vi "Color Table Generator.vi"() -> (0 "Color Map":u32[](array[colorbox])=[0, 15606540, 15541260, 15410444, 15345165, 15279629, 15214349, 15083534, 15018254, 14952974, 14822158, 14756622, 14691343, 14560527, 14495247, 14429968, 14364688, 14233616, 14168336, 14103056, 13972241, 13906961, 13841681, 13776146, 13645330, 13580050, 13514770, 13383954, 13318675, 13253395, 13122323, 13057044, 12991764, 12926484, 12795668, 12730388, 12664853, 12534037, 12468757, 12403478, 12338198, 12207382, 12141846, 12076566, 11945751, 11880471, 11815191, 11749912, 11618840, 11553560, 11488280, 11357464, 11292185, 11226905, 11096089, 11030554, 10965274, 10899994, 10769178, 10703898, 10638619, 10507547, 10442267, 10376988, 10311708, 10180892, 10115612, 10050076, 9919261, 9853981, 9788701, 9657886, 9592606, 9527070, 9461790, 9330974, 9265695, 9200415, 9069599, 9004064, 8938784, 8873504, 8742688, 8677408, 8612129, 8481313, 8415777, 8350498, 8219682, 8154402, 8089122, 8023842, 7892771, 7827491, 7762211, 7631396, 7566116, 7500836, 7435300, 7304484, 7239205, 7173925, 7043109, 6977830, 6912294, 6847014, 6716198, 6650918, 6585639, 6454823, 6389543, 6324008, 6193192, 6127912, 6062632, 5997352, 5866537, 5801001, 5801257, 5735978, 5736234, 5670954, 5671210, 5605674, 5605931, 5540651, 5540907, 5475628, 5475884, 5410348, 5410605, 5345327, 5345584, 5279793, 5279539, 5213748, 5213493, 5147703, 5147704, 5081913, 5081659, 5015868, 5015613, 4949823, 4949568, 4949314, 4883523, 4883268, 4817734, 4817479, 4751688, 4751434, 4685643, 4685388, 4619598, 4619343, 4553552, 4553298, 4487763, 4487508, 4421718, 4421463, 4355672, 4355418, 4289627, 4289372, 4223582, 4223327, 4157792, 4157538, 4091747, 4091492, 4091238, 4025447, 4025192, 3959402, 3959147, 3893357, 3893358, 3827567, 3827313, 3761522, 3761267, 3695477, 3695222, 3629431, 3629177, 3563386, 3563387, 3497597, 3497342, 3431551, 3431297, 3365506, 3365251, 3299461, 3299206, 3233415, 3233161, 3167626, 3167371, 3167117, 3101326, 3101071, 3035281, 3035026, 2969235, 2968981, 2903190, 2903192, 2837401, 2837146, 2771356, 2771101, 2705310, 2705056, 2639265, 2639010, 2573220, 2573221, 2507430, 2507176, 2441385, 2441130, 2375340, 2375085, 2309294, 2309040, 2308785, 2243250, 2242996, 2177205, 2176950, 2111160, 2110905, 2045114, 2044860, 1979069, 1978814, 1913280, 1913025, 1847235, 1846980, 1781189, 1780935, 1715144, 1714889, 1649099, 1648844, 1583309, 1583055, 1517264, 1517009, 1451219, 1450964, 16711680])   [LabVIEW 2013]
doc: "Color Table Generator.vi is a subVI called by Color Table Example.vi\n\nThis VI generates a color table based on the beginning, middle, and end RGB color combinations the user specifies. Using an XY graph and cursors, the user mixes red, green, and blue components to create the start, middle, and end color combinations for the color table."
panel:
  in  "Black and White":bool
  in  "Initial Color":cluster{dbl, dbl, dbl}(slide)={0.0, 0.0, 255.0} scale=0.0..255.0
  in  "Out of range below\n(color 0)":u32(colorbox)
  in  "Out of range above\n(color 255)":u32(colorbox)=16711680
  in  "Cancel":bool
  in  "Accept":bool
  in  "Final Color":cluster{dbl, dbl, dbl}(slide)={255.0, 0.0, 0.0} scale=0.0..255.0
  out "?":cluster{"Component array":u8[]}[](graph)=[{"Component array"=[0, 2, 4, 6, 8, 10, 12, 14, 16, 18, 20, 22, 24, 26, 28, 30, 32, 34, 36, 38, 40, 43, 45, 47, 49, 51, 53, 55, 57, 59, 61, 63, 65, 67, 69, 71, 73, 75, 77, 79, 81, 83, 85, 87, 89, 91, 93, 95, 97, 99, 101, 103, 105, 107, 109, 111, 113, 115, 117, 119, 121, 123, 125, 127, 130, 132, 134, 136, 138, 140, 142, 144, 146, 148, 150, 152, 154, 156, 158, 160, 162, 164, 166, 168, 170, 172, 174, 176, 178, 180, 182, 184, 186, 188, 190, 192, 194, 196, 198, 200, 202, 204, 206, 208, 210, 212, 215, 217, 219, 221, 223, 225, 227, 229, 231, 233, 235, 237, 239, 241, 243, 245, 247, 249, 251, 253, 255, 255, 255, 255, 255, 255, 255, 255, 255, 255, 255, 255, 255, 255, 255, 255, 255, 255, 255, 255, 255, 255, 255, 255, 255, 255, 255, 255, 255, 255, 255, 255, 255, 255, 255, 255, 255, 255, 255, 255, 255, 255, 255, 255, 255, 255, 255, 255, 255, 255, 255, 255, 255, 255, 255, 255, 255, 255, 255, 255, 255, 255, 255, 255, 255, 255, 255, 255, 255, 255, 255, 255, 255, 255, 255, 255, 255, 255, 255, 255, 255, 255, 255, 255, 255, 255, 255, 255, 255, 255, 255, 255, 255, 255, 255, 255, 255, 255, 255, 255, 255, 255, 255, 255, 255, 255, 255, 255, 255, 255, 255, 255, 255, 255, 255, 255, 255, 255, 255, 255, 255, 255, 255, 255, 255, 255, 255, 255]}, {"Component array"=[0, 2, 4, 6, 8, 10, 12, 14, 16, 18, 20, 22, 24, 26, 28, 30, 32, 34, 36, 38, 40, 41, 43, 45, 47, 49, 51, 53, 55, 57, 59, 61, 63, 65, 67, 69, 71, 73, 75, 77, 79, 81, 83, 85, 87, 89, 91, 93, 95, 97, 99, 101, 103, 105, 107, 109, 111, 113, 115, 117, 119, 121, 123, 125, 126, 128, 130, 132, 134, 136, 138, 140, 142, 144, 146, 148, 150, 152, 154, 156, 158, 160, 162, 164, 166, 168, 170, 172, 174, 176, 178, 180, 182, 184, 186, 188, 190, 192, 194, 196, 198, 200, 202, 204, 206, 208, 209, 211, 213, 215, 217, 219, 221, 223, 225, 227, 229, 231, 233, 235, 237, 239, 241, 243, 245, 247, 249, 247, 245, 243, 241, 239, 237, 235, 233, 231, 229, 227, 225, 224, 222, 220, 218, 216, 214, 212, 210, 208, 206, 204, 202, 200, 198, 196, 194, 192, 190, 188, 186, 184, 182, 180, 178, 176, 174, 173, 171, 169, 167, 165, 163, 161, 159, 157, 155, 153, 151, 149, 147, 145, 143, 141, 139, 137, 135, 133, 131, 129, 127, 125, 124, 122, 120, 118, 116, 114, 112, 110, 108, 106, 104, 102, 100, 98, 96, 94, 92, 90, 88, 86, 84, 82, 80, 78, 76, 75, 73, 71, 69, 67, 65, 63, 61, 59, 57, 55, 53, 51, 49, 47, 45, 43, 41, 39, 37, 35, 33, 31, 29, 27, 25, 24, 22, 20, 18, 16, 14, 12, 10, 8, 6, 4, 2, 0]}, {"Component array"=[255, 253, 251, 249, 247, 245, 243, 241, 239, 237, 235, 233, 231, 228, 226, 224, 222, 220, 218, 216, 214, 212, 210, 208, 206, 204, 202, 200, 198, 196, 194, 192, 190, 188, 186, 184, 182, 180, 177, 175, 173, 171, 169, 167, 165, 163, 161, 159, 157, 155, 153, 151, 149, 147, 145, 143, 141, 139, 137, 135, 133, 131, 129, 126, 124, 122, 120, 118, 116, 114, 112, 110, 108, 106, 104, 102, 100, 98, 96, 94, 92, 90, 88, 86, 84, 82, 80, 77, 75, 73, 71, 69, 67, 65, 63, 61, 59, 57, 55, 53, 51, 49, 47, 45, 43, 41, 39, 37, 35, 33, 31, 29, 26, 24, 22, 20, 18, 16, 14, 12, 10, 8, 6, 4, 2, 2, 2, 2, 2, 2, 2, 2, 2, 2, 2, 2, 2, 2, 2, 2, 2, 2, 2, 2, 2, 2, 2, 2, 2, 2, 2, 2, 2, 2, 2, 2, 2, 1, 1, 1, 1, 1, 1, 1, 1, 1, 1, 1, 1, 1, 1, 1, 1, 1, 1, 1, 1, 1, 1, 1, 1, 1, 1, 1, 1, 1, 1, 1, 1, 1, 1, 1, 1, 1, 1, 1, 1, 1, 1, 1, 1, 1, 1, 1, 1, 1, 1, 1, 1, 1, 1, 1, 1, 1, 1, 1, 1, 1, 1, 1, 1, 0, 0, 0, 0, 0, 0, 0, 0, 0, 0, 0, 0, 0, 0, 0, 0, 0, 0, 0, 0, 0, 0, 0, 0, 0, 0, 0, 0, 0, 0, 0, 0, 0]}]
  # "Use the two sliders and the cursors to define the color table."
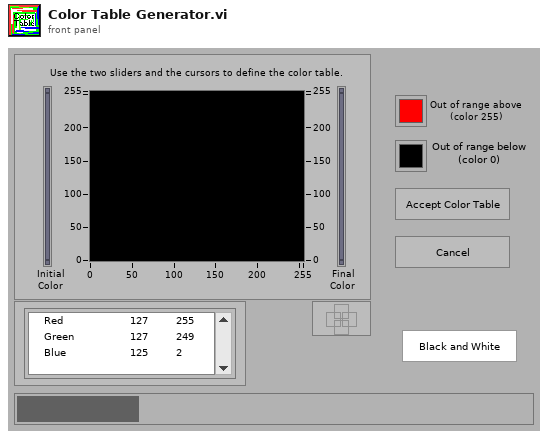
[diagram p1: front panel]
types:
  T1 = cluster{dbl, dbl, "Cursor.Cursor Y":dbl, "Cursor.Cursor X":dbl}
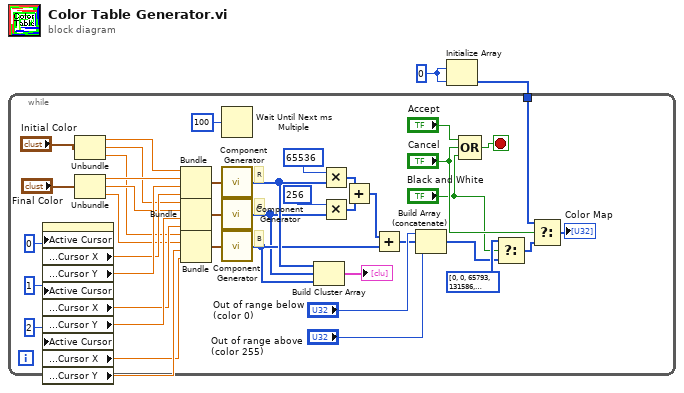
[diagram p0: block diagram]
diagram:
  w2 = u32 0
  n1 = Initialize Array(w2, w2) -> (w1:u32[])
  n2 = while {
    tunnel: w1 -> [w18]
    stop <- w19 stop-if-true
    # "B"
    # "G"
    # "R"
    n3 = property class="WFGraph (strict)"("Active Cursor"=0, "Active Cursor"=1, "Active Cursor"=2) -> ("Cursor.Cursor Position:Cursor X"=w39:dbl, "Cursor.Cursor Position:Cursor Y"=w40:dbl, "Cursor.Cursor Position:Cursor X"=w41:dbl, "Cursor.Cursor Position:Cursor Y"=w42:dbl, "Cursor.Cursor Position:Cursor X"=w43:dbl, "Cursor.Cursor Position:Cursor Y"=w44:dbl)  [unwired: 2 in, 2 out]
    n4 = Unbundle("Initial Color") -> (w33:dbl, w34:dbl, w35:dbl)
    n5 = Unbundle("Final Color") -> (w36:dbl, w37:dbl, w38:dbl)
    n6 = Bundle(w33, w36, "Cursor.Cursor Y"=w40, "Cursor.Cursor X"=w39) -> (w31:T1)  [unwired: 1 in]
    n7 = Bundle(w34, w37, "Cursor.Cursor Y"=w42, "Cursor.Cursor X"=w41) -> (w15:T1)  [unwired: 1 in]
    n8 = Bundle(w35, w38, "Cursor.Cursor Y"=w44, "Cursor.Cursor X"=w43) -> (w14:T1)  [unwired: 1 in]
    n9 = Wait Until Next ms Multiple(millisecond multiple=u32 100) -> ()  [unwired: 1 out]
    n10 = call "Component Generator.vi"("Component definition"=w31) -> ("Component array"=w27:u8[])
    n11 = call "Component Generator.vi"("Component definition"=w15) -> ("Component array"=w12:u8[])
    n12 = call "Component Generator.vi"("Component definition"=w14) -> ("Component array"=w13:u8[])
    n13 = Build Cluster Array(w27, w12, w13) -> (→"?":cluster{"Component array":u8[]}[])
    n14 = Multiply(x=u32 65536, y=w27) -> (x*y=w24:u32[])
    n15 = Multiply(x=u32 256, y=w12) -> (x*y=w23:u32[])
    n16 = Add(x=w24, y=w23) -> (x+y=w25:u32[])
    n17 = Add(x=w25, y=w13) -> (x+y=w9:u32[])
    n18 = Build Array (concatenate)("Out of range below\n(color 0)", w9, "Out of range above\n(color 255)") -> (w5:u32[])
    n19 = Compound Arithmetic op=OR("Accept", "Cancel", "Black and White") -> (w19:bool)
    n20 = Select(t=u32[] [0, 0, 65793, 131586, 197379, 263172, 328965, 394757, 395014, 460807, 526344, 592137, 657930, 723723, 789516, 855309, 921102, 986895, 1052688, 1118480, 1184273, 1184530, 1250323, 1316116, 1381909, 1447702, 1513495, 1579288, 1644825, 1710618, 1776410, 1842203, 1907996, 1973789, 1974046, 2039839, 2105632, 2171425, 2237218, 2303011, 2368804, 2434597, 2500389, 2566182, 2631975, 2697768, 2763305, 2763562, 2829355, 2895148, 2960941, 3026734, 3092527, 3158319, 3224112, 3289905, 3355698, 3421491, 3487284, 3553077, 3553334, 3619127, 3684920, 3750713, 3816249, 3882042, 3947835, 4013628, 4079421, 4145214, 4211007, 4276800, 4277057, 4342850, 4408643, 4474436, 4540228, 4606021, 4671814, 4737607, 4803400, 4869193, 4934730, 5000523, 5066316, 5066573, 5132366, 5198158, 5263951, 5329744, 5395537, 5461330, 5527123, 5592916, 5658709, 5724502, 5790295, 5856088, 5856345, 5922137, 5987674, 6053467, 6119260, 6185053, 6250846, 6316639, 6382432, 6448225, 6514018, 6579811, 6645603, 6645860, 6711653, 6777446, 6843239, 6909032, 6974825, 7040618, 7106155, 7171948, 7237741, 7303534, 7369326, 7435119, 7435376, 7501169, 7566962, 7632755, 7698548, 7764341, 7830134, 7895927, 7961721, 8027514, 8093563, 8159356, 8290685, 8356478, 8422271, 8488064, 8553857, 8619650, 8685444, 8751237, 8817030, 8882823, 9014152, 9079945, 9145994, 9211787, 9277580, 9343373, 9409167, 9474960, 9540753, 9606546, 9737875, 9803668, 9869461, 9935254, 10001047, 10066840, 10132890, 10198683, 10264476, 10330269, 10396062, 10527391, 10593184, 10658977, 10724770, 10790564, 10856357, 10922150, 10987943, 11053736, 11119785, 11251114, 11316907, 11382700, 11448493, 11514287, 11580080, 11645873, 11711666, 11777459, 11843252, 11974581, 12040374, 12106167, 12172216, 12238010, 12303803, 12369596, 12435389, 12501182, 12566975, 12632768, 12764097, 12829890, 12895683, 12961477, 13027270, 13093063, 13158856, 13224905, 13290698, 13356491, 13487820, 13553613, 13619406, 13685200, 13750993, 13816786, 13882579, 13948372, 14014165, 14079958, 14211287, 14277336, 14343130, 14408923, 14474716, 14540509, 14606302, 14672095, 14737888, 14803681, 14869474, 15000803, 15066597, 15132390, 15198183, 15264232, 15330025, 15395818, 15461611, 15527404, 15593197, 15724526, 15790320, 15856113, 15921906, 15987699, 16053492, 16119285, 16185078, 16251127, 16316920, 16448249, 16514043, 16579836, 16645629, 16711422, 16777215, 16711680] ("Black and White"), s="Black and White", f=w5) -> (s? t:f=w4:u32[])
    n21 = Select(t=w18, s="Cancel", f=w4) -> (s? t:f=→"Color Map":u32[])
  }
